vi "Measure Voltage Drop.vi"(0 "Automation Refnum in":T2, 5 "RLY12V_MEAS":T3, 7 "SSC":T8[](array[typedef]), 9 "Relay TSM in":T1, 11 "error in (no error)":errorcluster) -> (4 "Voltage Measurements (V)":dbl[](array[numeric]), 15 "error out":errorcluster)   [LabVIEW 2019]
uses:
  Common/Instrument Control/DAQmx/Pin Map/SSC DAQmx.ctl
  <vilib>/NI_TestStand_SemiconductorModule/NI_TestStand_Semiconductor_Module.lvlibp/PinMap/General/SemiconductorModuleContext.ctl
  Common/Instrument Control/DCPower/TSM/TSM SSC DCPower.ctl
  <vilib>/NI_TestStand_SemiconductorModule/NI_TestStand_Semiconductor_Module.lvlibp/PinMap/PinQueryContext/MultiplePinMultipleSessionQueryContext/MultiplePinMultipleSessionQueryContext.lvclass
  Common/Instrument Control/DCPower/SSC DCPower/SSC DCPower.ctl
  Common/Instrument Control/Shared SubVIs/TSM Pin Abstraction/TSM Pin Information.ctl
  Common/Instrument Control/Shared SubVIs/TSM Pin Abstraction/TSM Pin Type Identifier.ctl
  Common/Instrument Control/Shared SubVIs/TSM Pin Abstraction/TSM Expanded Pin Information.ctl
  Common/Instrument Control/Relay/Pin Map/TSM Relay.ctl
  <vilib>/NI_TestStand_SemiconductorModule/NI_TestStand_Semiconductor_Module.lvlibp/1abvi3w/instr.lib/niSwitch/niswitch.llb/niSwitch Relay Action.ctl
  <vilib>/NI_TestStand_SemiconductorModule/NI_TestStand_Semiconductor_Module.lvlibp/PinMap/Relay Driver/ControlRelay(s).vi
  <vilib>/NI_TestStand_SemiconductorModule/NI_TestStand_Semiconductor_Module.lvlibp/PinMap/Relay Driver/ControlRelaysSingleAction.vi
  Common/Instrument Control/DCPower/SSC DCPower/SSC DCPower Measure.vi
  <vilib>/NI_TestStand_SemiconductorModule/NI_TestStand_Semiconductor_Module.lvlibp
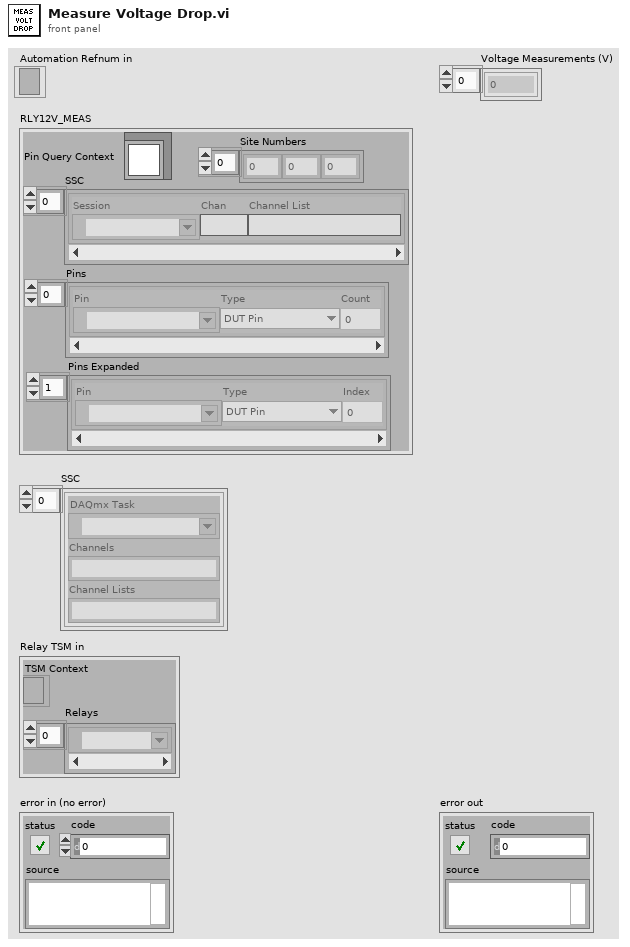
[diagram p1: front panel]
types:
  T1 = typedef "TSM Relay.ctl" = cluster{"TSM Context":T2, "Relays":tag[]}
  T2 = typedef "NI_TestStand_Semiconductor_Module.lvlibp/SemiconductorModuleContext.ctl" = refnum<k7>
  T3 = typedef "TSM SSC DCPower.ctl" = cluster{"Pin Query Context":refnum<class "MultiplePinMultipleSessionQueryContext.lvclass">, "SSC":T4[], "Site Numbers":i32[], "Pins":T5[], "Pins Expanded":T7[]}
  T4 = typedef "SSC DCPower.ctl" = cluster{"Session":refnum<k15>, "Chan":string, "Channel List":string}
  T5 = typedef "TSM Pin Information.ctl" = cluster{"Pin":tag, "Type":T6, "Count":i32}
  T6 = typedef "TSM Pin Type Identifier.ctl" = enum8{"DUT Pin", "System Pin", "Pin Group", "Not Determined"}
  T7 = typedef "TSM Expanded Pin Information.ctl" = cluster{"Pin":tag, "Type":T6, "Index":i32}
  T8 = typedef "SSC DAQmx.ctl" = cluster{"DAQmx Task ":refnum<k21>, "Channels":string, "Channel Lists":string}
  T9 = typedef "NI_TestStand_Semiconductor_Module.lvlibp/niSwitch Relay Action.ctl" = i32
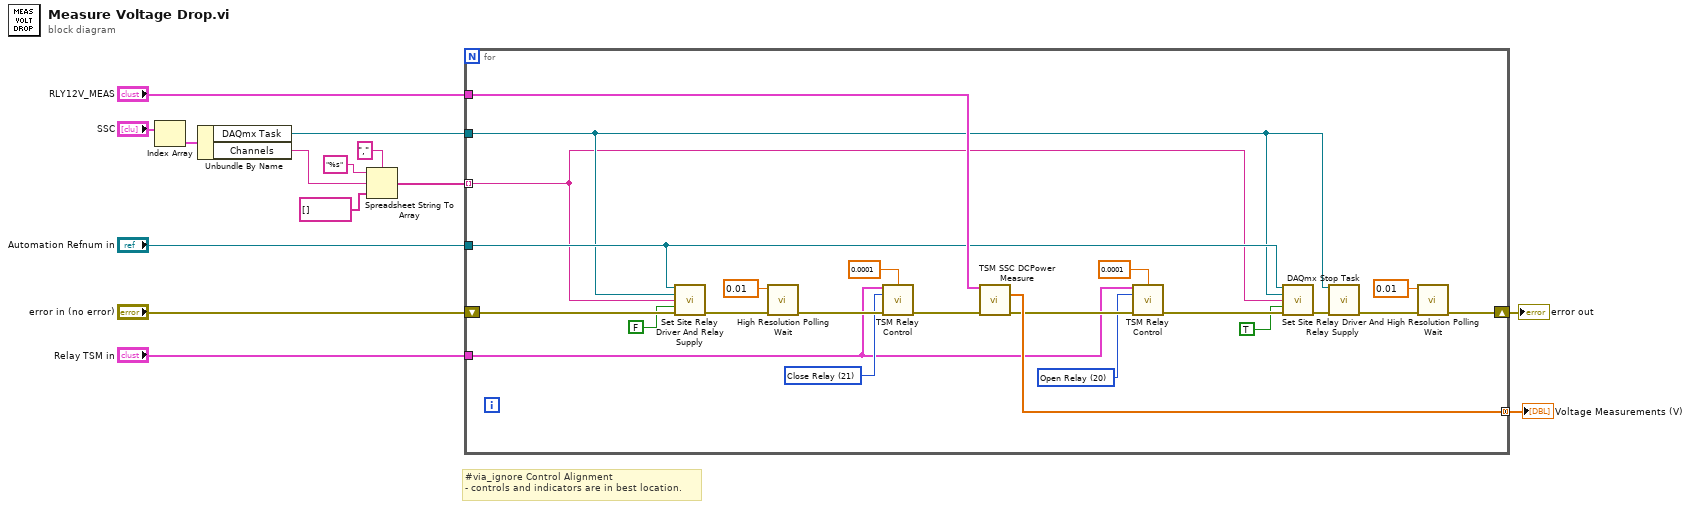
[diagram p0: block diagram]
diagram:
  # "#via_ignore Control Alignment\n- controls and indicators are in best location."
  n1 = Index Array(array="SSC") -> (element=w7:T8)  [unwired: 1 in]
  n2 = Unbundle By Name(w7) -> ("DAQmx Task"=w6:refnum<k21>, "Channels"=w2:string)
  n3 = Spreadsheet String To Array(delimiter (Tab)=",", format string="%s", spreadsheet string=w2, array type (2D Dbl)=string[] [] ("format string")) -> (array=w1:string[])
  n4 = for {
    tunnel: "Automation Refnum in" -> [w34]
    shift-right: [w28] -> w13
    shift-left: "error in (no error)" -> [w37]
    tunnel: "RLY12V_MEAS" -> [w35]
    tunnel: [w31] -> w11 mode=concatenating
    tunnel: "Relay TSM in" -> [w23]
    tunnel: w6 -> [w27]
    tunnel: w1 -> [w15] mode=indexing
    w25 = T9 20 items=["Open Relay"=20, "Close Relay"=21] ("Relay Action")
    w30 = T9 21 items=["Open Relay"=20, "Close Relay"=21] ("Relay Action")
    n5 = call "Set Site Relay Driver And Relay Supply.vi"("TSM Context"=w34, "DAQmx Task"=w27, "SSC.Channels"=w15, "State (F:Enable)"=FALSE, "error in"=w37) -> ("error out"=w29:errorcluster)  [unwired: 10 in]
    n6 = call <vilib>:"High Resolution Polling Wait.vi"("error in (no error)"=w29, "seconds to wait"=0.01) -> ("error out"=w33:errorcluster)  [unwired: 9 in]
    n7 = call "TSM Relay Control.vi"("Relay TSM in"=w23, "Settling Time (s)"=0.0001, "Relay Action"=w30, "error in"=w33) -> ("error out"=w32:errorcluster)  [unwired: 11 in]
    n8 = call "TSM SSC DCPower Measure.vi"("DCPower TSM in"=w35, "error in"=w32) -> ("Voltage Measurements (V)"=w31:dbl[], "error out"=w26:errorcluster)  [unwired: 10 in, 2 out]
    n9 = call "TSM Relay Control.vi"("Relay TSM in"=w23, "Settling Time (s)"=0.0001, "Relay Action"=w25, "error in"=w26) -> ("error out"=w24:errorcluster)  [unwired: 11 in]
    n10 = call "Set Site Relay Driver And Relay Supply.vi"("TSM Context"=w34, "DAQmx Task"=w27, "SSC.Channels"=w15, "State (F:Enable)"=TRUE, "error in"=w24) -> ("error out"=w19:errorcluster)  [unwired: 10 in]
    n11 = call <vilib>:"DAQmx Stop Task.vi"("task/channels in"=w27, "error in"=w19) -> ("error out"=w16:errorcluster)  [unwired: 12 in, 1 out]
    n12 = call <vilib>:"High Resolution Polling Wait.vi"("error in (no error)"=w16, "seconds to wait"=0.01) -> ("error out"=w28:errorcluster)  [unwired: 9 in]
  }
  "error out" <- w13
  "Voltage Measurements (V)" <- w11
